vi "get_info.vi"(8 "error in (no error)":errorcluster, 11 "Connection in":refnum<class "Connection.lvclass">) -> (0 "error out":errorcluster, 2 "info.":string, 3 "Connection out":refnum<class "Connection.lvclass">)   [LabVIEW 2019, in "Socket API.lvlib" / "Connection.lvclass"]
uses:
  Connection.lvclass
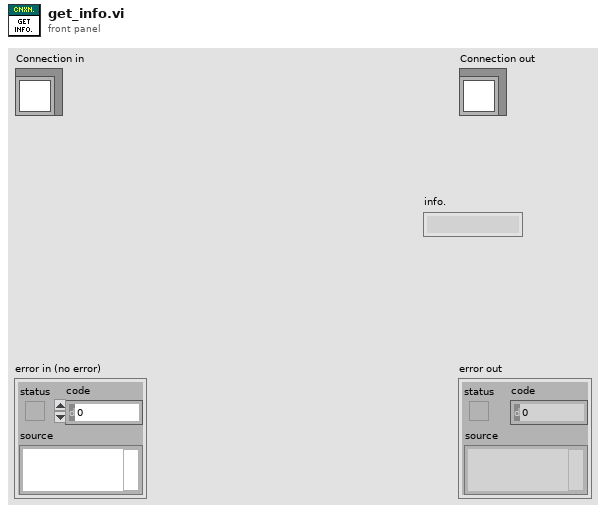
[diagram p1: front panel]
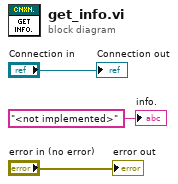
[diagram p0: block diagram]
diagram:
  "error out" <- "error in (no error)"
  "Connection out" <- "Connection in"
  "info." <- "<not implemented>" ("info.")
